vi "NF WF1973_74 SEQ Rec.vi"(8 "error in (no error)":errorcluster caption="Error IN", 9 "File No.(1)":i32=1 min=1 max=10 step=1, 10 "Set No.(Input)":u16(ring) items=["Input", "Minimum", "Maximum"], 11 "VISAsession":refnum<visa-resource-name>) -> (0 "error out":errorcluster caption="Error OUT", 3 "CopyVISAsession":refnum<visa-resource-name>)   [LabVIEW 2010]
panel:
  # "Choose\nInput"
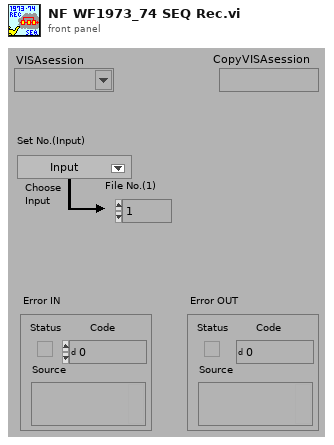
[diagram p1: front panel]
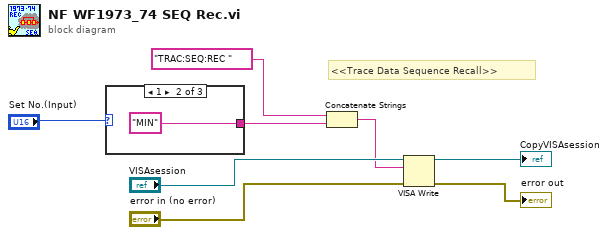
[diagram p0: block diagram]
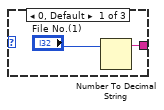
[diagram p2: hidden frame]
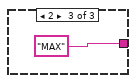
[diagram p3: hidden frame]
diagram:
  # "<<Trace Data Sequence Recall>>"
  n1 = case shown="1" "Set No.(Input)" {
    tunnel: [w9 "MIN" "MAX"] -> w3
    frame 0, Default {
      n2 = Number To Decimal String(number="File No.(1)") -> (decimal integer string=w9:string)  [unwired: 1 in]
    }
    frame 1 {
    }
    frame 2 {
    }
  }
  n3 = Concatenate Strings("TRAC:SEQ:REC ", w3) -> (w2:string)
  n4 = VISA Write(VISA resource name="VISAsession", write buffer=w2, error in (no error)="error in (no error)") -> (VISA resource name out=→"CopyVISAsession":refnum<visa-resource-name>, error out=→"error out":errorcluster)  [unwired: 1 out]
